vi "close.vi"(8 "error in (no error)":errorcluster, 11 "ScopeNi in":refnum<class "ScopeNi.lvclass">) -> (0 "error out":errorcluster)   [LabVIEW 2023, in "ScopeNi.lvclass"]
doc: "Close the Instrument Reference"
uses:
  ScopeNi.lvclass
  ScopeNi.lvclass/ScopeNi.ctl
  Scope.lvclass
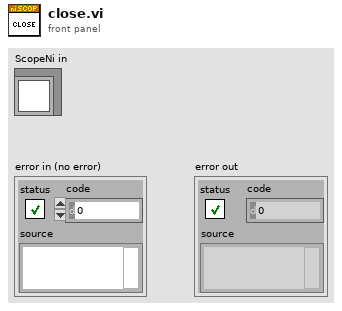
[diagram p1: front panel]
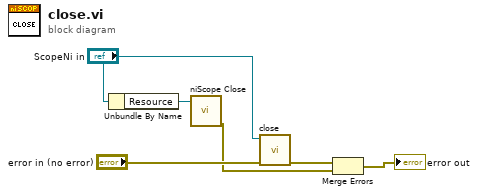
[diagram p0: block diagram]
diagram:
  n1 = Unbundle By Name("ScopeNi in") -> ("Resource"=w3:refnum<k15>)
  n2 = call <instrlib>:"niScope Close.vi"("instrument handle"=w3) -> ("error out"=w1:errorcluster)  [unwired: 14 in]
  n3 = call-parent "close.vi"("error in (no error)"="error in (no error)", "Instrument in"="ScopeNi in") -> ("error out"=w6:errorcluster)  [unwired: 9 in]
  n4 = Merge Errors(w6, w1) -> (→"error out":errorcluster)
